vi "Error Codes.vi"(6 "Parameter":string, 7 "Error":T1, 8 "error in (no error)":errorcluster, 9 "Signal Type":string, 10 "Module/Signal Name":string, 11 "Module/Signal Resource":string) -> (0 "error out":errorcluster)   [LabVIEW 2025, in "VI.lvclass"]
doc: "Create Error Cluster with Specifics."
uses:
  VI.lvclass
  Error Codes.ctl
  VI.lvclass/VI.ctl
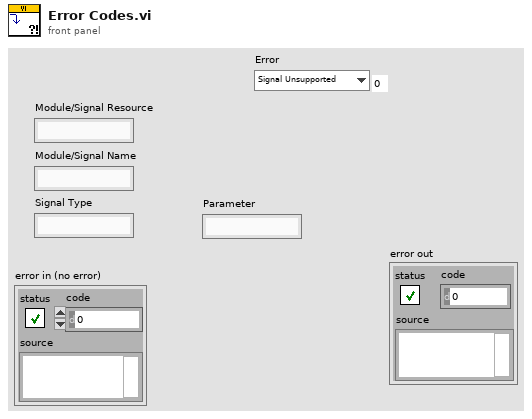
[diagram p1: front panel]
types:
  T1 = typedef "VI.lvclass/Error Codes.ctl" = enum16{"Signal Unsupported", "Module Unsupported", "Parameter Unsupported", "Signal Code Gen Error", "Module Code Gen Error", "Cleanup Code Error", "Signal Direction Mismatch", "Signal Type Mismatch", "Module Channel Number Mismatch", "Minimum Channels Mismatch"}
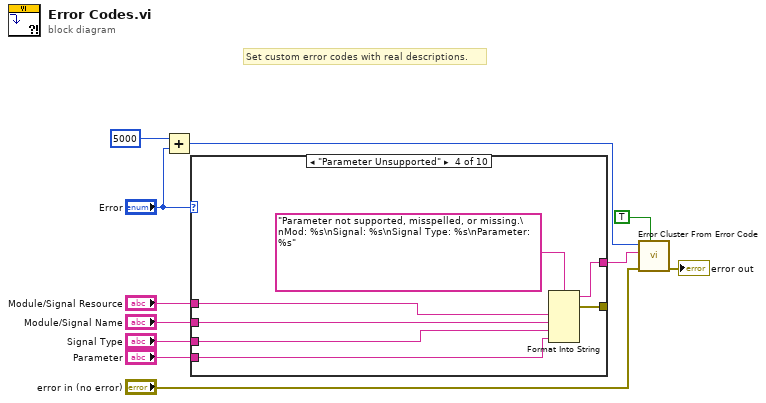
[diagram p0: block diagram]
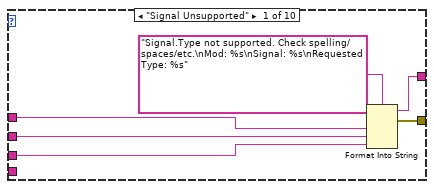
[diagram p2: hidden frame]
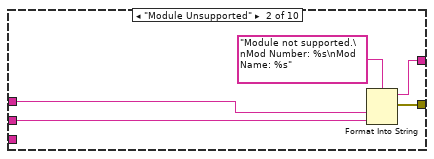
[diagram p3: hidden frame]
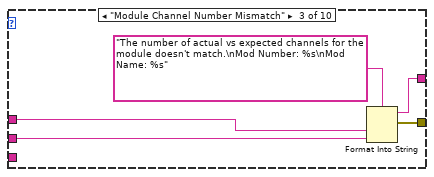
[diagram p4: hidden frame]
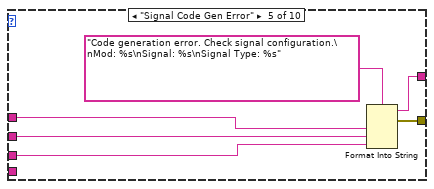
[diagram p5: hidden frame]
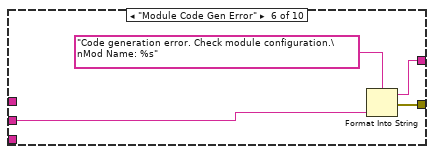
[diagram p6: hidden frame]
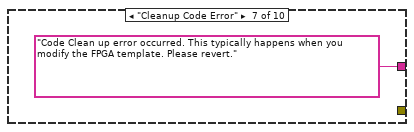
[diagram p7: hidden frame]
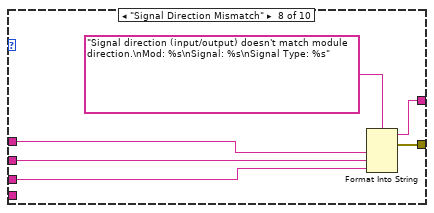
[diagram p8: hidden frame]
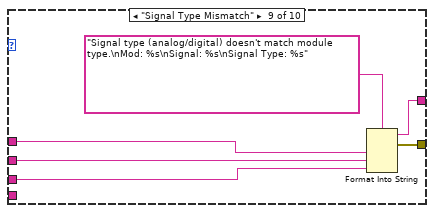
[diagram p9: hidden frame]
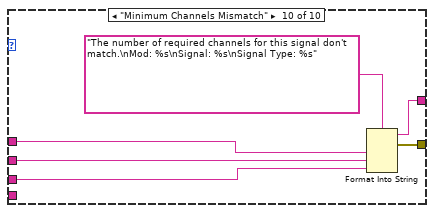
[diagram p10: hidden frame]
diagram:
  # "Set custom error codes with real descriptions."
  n1 = Add(x=5000, y="Error") -> (x+y=w4:i32)
  n2 = case shown="\"Parameter Unsupported\"" "Error" {
    tunnel: [w16 w21 w26 w33 w39 w43 "Code Clean up error occurred. This typically happens when you modify the FPGA template. Please revert." ("error message (\"\")") w50 w56 w62] -> w10
    tunnel: [w15 w20 w25 w32 w38 w42 _ w49 w55 w61] -> _
    tunnel: "Module/Signal Name" -> [w14 w18 w23 w30 w36 w41 _ w47 w53 w59]
    tunnel: "Module/Signal Resource" -> [w13 w19 w24 w31 w37 _ _ w48 w54 w60]
    tunnel: "Signal Type" -> [w12 _ _ w29 w35 _ _ w46 w52 w58]
    tunnel: "Parameter" -> [_ _ _ w28 _ _ _ _ _ _]
    frame "Signal Unsupported" {
      n3 = Format Into String(format string="Signal.Type not supported. Check spelling/spaces/etc.\nMod: %s\nSignal: %s\nRequested Type: %s" ("error message (\"\")"), w13, w14, w12) -> (resulting string=w16:string, error out=w15:errorcluster)  [unwired: 2 in]
    }
    frame "Module Unsupported" {
      n4 = Format Into String(format string="Module not supported.\nMod Number: %s\nMod Name: %s" ("error message (\"\")"), w19, w18) -> (resulting string=w21:string, error out=w20:errorcluster)  [unwired: 2 in]
    }
    frame "Module Channel Number Mismatch" {
      n5 = Format Into String(format string="The number of actual vs expected channels for the module doesn't match.\nMod Number: %s\nMod Name: %s" ("error message (\"\")"), w24, w23) -> (resulting string=w26:string, error out=w25:errorcluster)  [unwired: 2 in]
    }
    frame "Parameter Unsupported" {
      n6 = Format Into String(format string="Parameter not supported, misspelled, or missing.\nMod: %s\nSignal: %s\nSignal Type: %s\nParameter: %s" ("error message (\"\")"), w31, w30, w29, w28) -> (resulting string=w33:string, error out=w32:errorcluster)  [unwired: 2 in]
    }
    frame "Signal Code Gen Error" {
      n7 = Format Into String(format string="Code generation error. Check signal configuration.\nMod: %s\nSignal: %s\nSignal Type: %s" ("error message (\"\")"), w37, w36, w35) -> (resulting string=w39:string, error out=w38:errorcluster)  [unwired: 2 in]
    }
    frame "Module Code Gen Error" {
      n8 = Format Into String(format string="Code generation error. Check module configuration.\nMod Name: %s" ("error message (\"\")"), w41) -> (resulting string=w43:string, error out=w42:errorcluster)  [unwired: 2 in]
    }
    frame "Cleanup Code Error" {
    }
    frame "Signal Direction Mismatch" {
      n9 = Format Into String(format string="Signal direction (input/output) doesn't match module direction.\nMod: %s\nSignal: %s\nSignal Type: %s" ("error message (\"\")"), w48, w47, w46) -> (resulting string=w50:string, error out=w49:errorcluster)  [unwired: 2 in]
    }
    frame "Signal Type Mismatch" {
      n10 = Format Into String(format string="Signal type (analog/digital) doesn't match module type.\nMod: %s\nSignal: %s\nSignal Type: %s" ("error message (\"\")"), w54, w53, w52) -> (resulting string=w56:string, error out=w55:errorcluster)  [unwired: 2 in]
    }
    frame "Minimum Channels Mismatch" {
      n11 = Format Into String(format string="The number of required channels for this signal don't match.\nMod: %s\nSignal: %s\nSignal Type: %s" ("error message (\"\")"), w60, w59, w58) -> (resulting string=w62:string, error out=w61:errorcluster)  [unwired: 2 in]
    }
  }
  n12 = call <vilib>:"Error Cluster From Error Code.vi"("show call chain? (False)"=TRUE, "error in (no error)"="error in (no error)", "error message (\"\")"=w10, "error code (0)"=w4) -> ("error out"=→"error out":errorcluster)  [unwired: 5 in]
